vi "Check Eaten Fruit.vi"(0 "Board Game in":refnum<class "Board Game.lvclass">, 2 "Packed refs":T1, 11 "error in (no error)":errorcluster) -> (4 "Board Game out":refnum<class "Board Game.lvclass">, 15 "error out":errorcluster)   [LabVIEW 2021, in "Board Game.lvclass"]
uses:
  Board Game.lvclass
  Application/Packed Refs.ctl
  GameEl_class/private/Enum Direction.ctl
  Board Game.lvclass/Board Game.ctl
  GameEl_class/GameEl.lvclass/GameEl.ctl
  Imposible_Snake_v2/LVApp/Modules/Sound Manager/Typedefs/Sound Effects.ctl
  <vilib>/numeric/Random Number (Range) DBL.vi
  GameEl_class/Read position.vi
  Snake_class/Snake.lvclass
  C:/Users/poche/Programs/LabVIEW/imposible snake/GameEl_class/GameEl.lvclass
  Fruit_class/Fruit.lvclass
  GameEl_class/GameEl.lvclass
  Imposible_Snake_v2/LVApp/Modules/Sound Manager/Sound Manager.lvlib
  Application/Game.lvclass
panel:
  out "Eaten Fruit?":bool
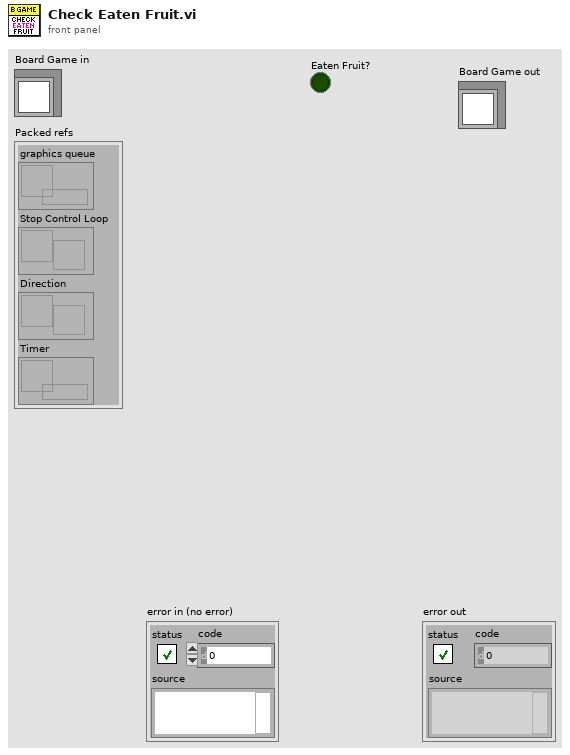
[diagram p1: front panel]
types:
  T1 = typedef "Game.lvclass/Packed Refs.ctl" = cluster{"graphics queue":refnum<queue>, "Stop Control Loop":refnum<user-event>, "Direction":refnum<notifier>, "Timer":refnum<data-value>}
  T2 = typedef "Sound Manager.lvlib/Sound Effects.ctl" = enum16{"Bomb In", "Bomb Out", "Bomb Touched", "Game Over", "Victory", "Eat", "10 Fruits", "Eat2", "Eat3", "Eat4", "MaxShield", "Shield", "10p", "Grape In", "Grape Out", "20p", "30p", "40p", "50p", "60p", "70p", "80p", "90p", "100p", "All shields cracked", "Mouse In", "Mouse Out", "Mouse Eaten", "Grape Eaten", "States Recover", "Broken Shield", "Bonus", "Happy Time", "explode", "Game over musica", "Back Music", "Shield Catch", "Evil lough", "Cricket In", "Cricket eaten", "Lets Go", "Jump1", "Jump2", "Jump3", "Unstoppable", "Troll Music", "winner", "menu"}
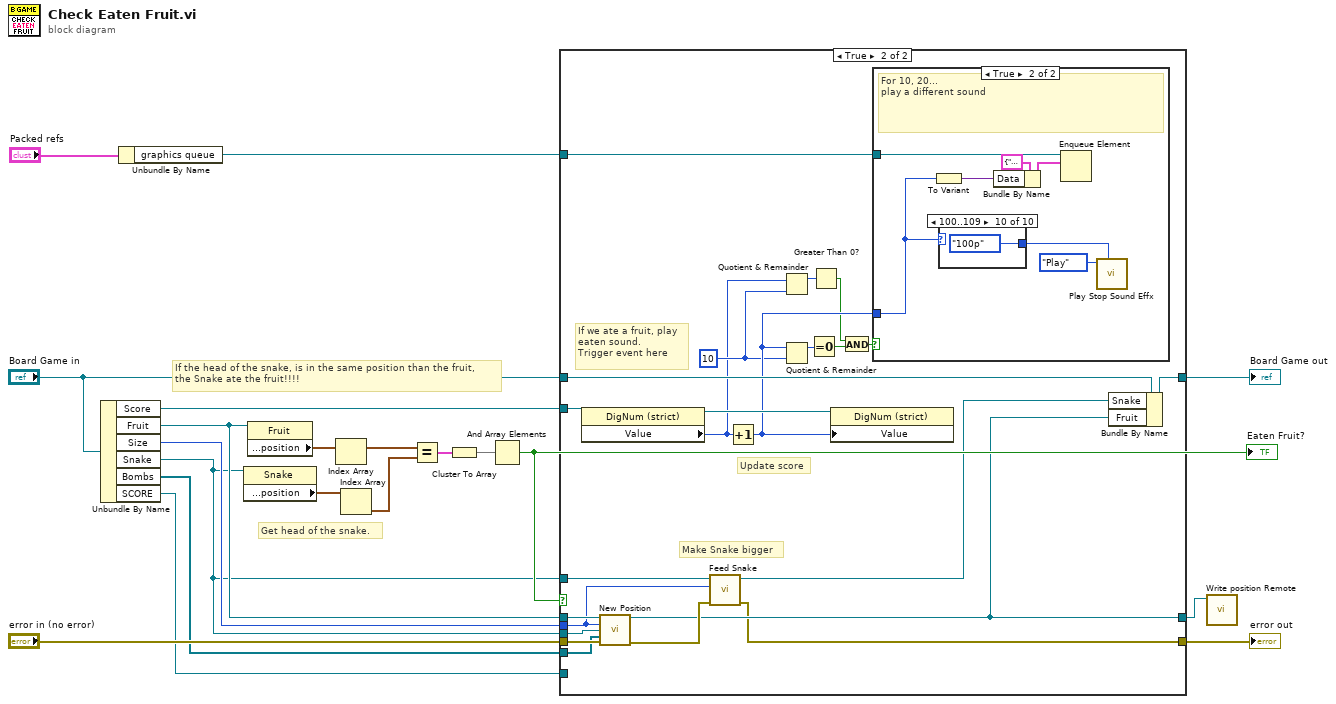
[diagram p0: block diagram]
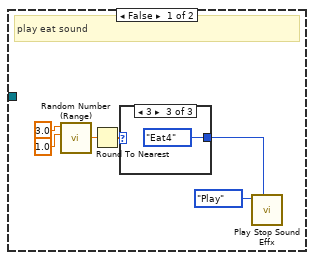
[diagram p3: hidden frame]
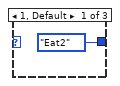
[diagram p4: hidden frame]
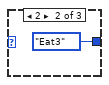
[diagram p5: hidden frame]
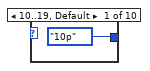
[diagram p6: hidden frame]
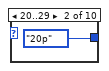
[diagram p7: hidden frame]
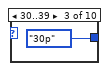
[diagram p8: hidden frame]
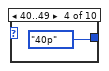
[diagram p9: hidden frame]
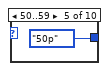
[diagram p10: hidden frame]
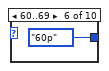
[diagram p11: hidden frame]
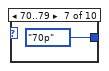
[diagram p12: hidden frame]
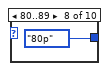
[diagram p13: hidden frame]
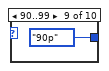
[diagram p14: hidden frame]
diagram:
  # "If the head of the snake, is in the same position than the fruit, \nthe Snake ate the fruit!!!!"
  # "Get head of the snake."
  n1 = Unbundle By Name("Board Game in") -> ("Score"=w8:refnum<vi>, "Fruit"=w13:refnum<class "Fruit.lvclass">, "Size"=w12:u16, "Snake"=w7:refnum<class "Snake.lvclass">, "Bombs"=w4:refnum<class "Bomb.lvclass">[], "SCORE"=w3:refnum<vi>)
  n2 = Unbundle By Name("Packed refs") -> ("graphics queue"=w5:refnum<queue>)
  n3 = property class="Snake"(reference=w7) -> ("SubVIs:DataAccess:position"=w20:cluster{"x":dbl, "y":dbl}[])  [unwired: 1 in, 2 out]
  n4 = property class="Fruit"(reference=w13) -> ("SubVIs:DataAccess:position"=w19:cluster{"x":dbl, "y":dbl}[])  [unwired: 1 in, 2 out]
  n5 = Index Array(array=w19) -> (element=w2:cluster{"x":dbl, "y":dbl})  [unwired: 1 in]
  n6 = Index Array(array=w20) -> (element=w18:cluster{"x":dbl, "y":dbl})  [unwired: 1 in]
  n7 = Equal?(x=w2, y=w18) -> (x = y?=w17:cluster{"x":bool, "y":bool})
  n8 = Cluster To Array(cluster=w17) -> (array=w16:bool[])
  n9 = And Array Elements(Boolean array=w16) -> (logical AND=w11:bool)
  "Eaten Fruit?" <- w11
  n10 = case shown="True" w11 {
    tunnel: "error in (no error)" -> [w23 w46]
    tunnel: [w23 w29] -> w14
    tunnel: w13 -> [w21 w45]
    tunnel: w12 -> [_ w36]
    tunnel: w7 -> [_ w44]
    tunnel: "Board Game in" -> [w22 w43]
    tunnel: [w22 w42] -> w9
    tunnel: w8 -> [_ w41]
    tunnel: w7 -> [_ w39]
    tunnel: w3 -> [_ _]
    tunnel: w5 -> [_ w33]
    tunnel: w4 -> [_ w32]
    tunnel: [w21 w31] -> w1
    frame False {
    }
    frame True {
      w28 = u16 10 ("y")
      # "If we ate a fruit, play \neaten sound. \nTrigger event here"
      # "Make Snake bigger"
      # "Update score"
      n11 = property class="DigNum (strict)"(reference=w41) -> (reference out=w40:refnum<vi>, "Value"=w27:u16)  [unwired: 1 in, 1 out]
      n12 = call "New Position.vi"("Fruit in"=w45, "B Game Size"=w36, "Snake"=w44, "Bomb"=w32, "error in (no error)"=w46) -> ("Fruit out"=w31:refnum<class "Fruit.lvclass">, "error out"=w37:errorcluster)  [unwired: 8 in, 1 out]
      n13 = call "Feed Snake.vi"("error in (no error)"=w37, "Size"=w36, "Snake in"=w39) -> ("error out"=w29:errorcluster, "Snake out"=w38:refnum<class "Snake.lvclass">)  [unwired: 7 in]
      n14 = Increment(x=w27) -> (x+1=w30:u16)
      n15 = Quotient & Remainder(x=w27, y=w28) -> (x-y*floor(x/y)=w26:u16)  [unwired: 1 out]
      n16 = Quotient & Remainder(x=w30, y=w28) -> (x-y*floor(x/y)=w35:u16)  [unwired: 1 out]
      n17 = Equal To 0?(x=w35) -> (x = 0?=w34:bool)
      n18 = Greater Than 0?(x=w26) -> (x > 0?=w24:bool)
      n19 = property class="DigNum (strict)"(reference=w40, "Value"=w30) -> ()  [unwired: 1 in, 2 out]
      n20 = And(x=w24, y=w34) -> (x .and. y?=w25:bool)
      n21 = case shown="True" w25 {
        tunnel: w33 -> [_ w62]
        tunnel: w30 -> [_ w58]
        frame False {
          # "play eat sound"
          n22 = call-poly <vilib>:"Random Number (Range).vi"("lower bound (0)"=1.0 ("Low"), "upper bound (100)"=3.0 ("High")) -> ("number"=w50:dbl)  [unwired: 9 in]
          n23 = Round To Nearest(number=w50) -> (nearest integer value=w49:dbl)
          n24 = case shown="3" w49 {
            tunnel: [Sound_Effects."Eat2" ("Sound Effect") Sound_Effects."Eat3" ("Sound Effect") Sound_Effects."Eat4" ("Sound Effect")] -> w47
            frame 1, Default {
            }
            frame 2 {
            }
            frame 3 {
            }
          }
          n25 = call "Play Stop Sound Effx.vi"("Sound Effect"=w47, "Function"=enum16{"Play", "Stop"}."Play") -> ()  [unwired: 9 in, 1 out]
        }
        frame True {
          # "For 10, 20...\nplay a different sound"
          n26 = To Variant(anything=w58) -> (Variant=w59:variant)
          n27 = case shown="100..109" w58 {
            tunnel: [Sound_Effects."10p" ("Sound Effect") Sound_Effects."20p" ("Sound Effect") Sound_Effects."30p" ("Sound Effect") Sound_Effects."40p" ("Sound Effect") Sound_Effects."50p" ("Sound Effect") Sound_Effects."60p" ("Sound Effect") Sound_Effects."70p" ("Sound Effect") Sound_Effects."80p" ("Sound Effect") Sound_Effects."90p" ("Sound Effect") Sound_Effects."100p" ("Sound Effect")] -> w56
            frame 10..19, Default {
            }
            frame 20..29 {
            }
            frame 30..39 {
            }
            frame 40..49 {
            }
            frame 50..59 {
            }
            frame 60..69 {
            }
            frame 70..79 {
            }
            frame 80..89 {
            }
            frame 90..99 {
            }
            frame 100..109 {
            }
          }
          n28 = Bundle By Name(cluster=cluster{"Message":string, "Data":variant} {"Message"="10 Points", "Data"=variant} ("element"), "Data"=w59) -> (w60:cluster{"Message":string, "Data":variant})
          n29 = Enqueue Element(queue=w62, element=w60) -> ()  [unwired: 2 in, 3 out]
          n30 = call "Play Stop Sound Effx.vi"("Sound Effect"=w56, "Function"=enum16{"Play", "Stop"}."Play") -> ()  [unwired: 9 in, 1 out]
        }
      }
      n31 = Bundle By Name(cluster=w43, "Snake"=w38, "Fruit"=w31) -> (w42:refnum<class "Board Game.lvclass">)
    }
  }
  "error out" <- w14
  "Board Game out" <- w9
  n32 = call "Write position Remote.vi"("GameEl in"=w1) -> ()  [unwired: 10 in, 1 out]
